vi "1D_array_rolling_avg.vi"(2 "N":i32=3, 3 "orig array":dbl[](array[numeric])=[0.0, 1.0, 2.0, 3.0, 4.0, 5.0, 6.0, 7.0, 8.0, 9.0]) -> (1 "moving centered avg":dbl[](array[numeric])=[0.5, 1.0, 2.0, 3.0, 4.0, 5.0, 6.0, 7.0, 8.0, 8.5])   [LabVIEW 2022 SP3]
uses:
  <vilib>/Analysis/baseanly.llb/Mean (DBL).vi
  <vilib>/Analysis/NI_AALBase.lvlib
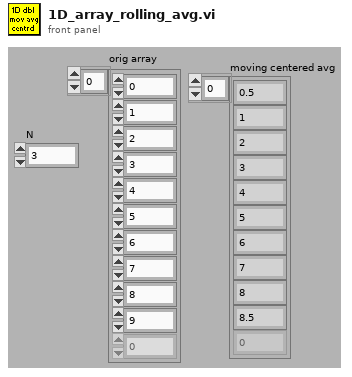
[diagram p1: front panel]
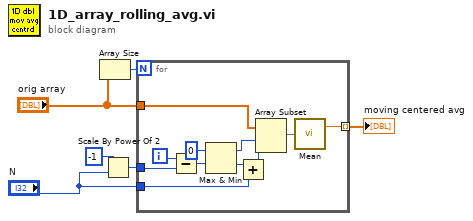
[diagram p0: block diagram]
diagram:
  n1 = Array Size(array="orig array") -> (size(s)=w2:i32)
  n2 = Scale By Power Of 2(n=-1, x="N") -> (x*2^n=w5:i32)
  n3 = for {
    N: w2 -> [_]
    tunnel: w5 -> [w15]
    tunnel: "N" -> [w11]
    tunnel: [w17] -> w4 mode=indexing
    tunnel: "orig array" -> [w7]
    i -> [w16]
    n4 = Subtract(x=w16, y=w15) -> (x-y=w14:i32)
    n5 = Max & Min(x=0, y=w14) -> (max(x,y)=w12:i32, min(x,y)=w8:i32)
    n6 = Add(x=w8, y=w11) -> (x+y=w9:i32)
    n7 = Array Subset(array=w7, index=w12, length=w9) -> (w10:dbl[])
    n8 = call-poly <vilib>:"Mean.vi"("X"=w10) -> ("mean"=w17:dbl)  [unwired: 1 out]
  }
  "moving centered avg" <- w4
